vi "界面.vi"() -> ()   [LabVIEW 2021]
uses:
  <vilib>/Utility/file.llb/Write Delimited Spreadsheet (string).vi
panel:
  out "回答框":string
  in  "词数":dbl(slide)=50.38167938931298 scale=0.0..200.0
  in  "空白按钮":bool
  in  "发送":bool
  in  "输入框":string
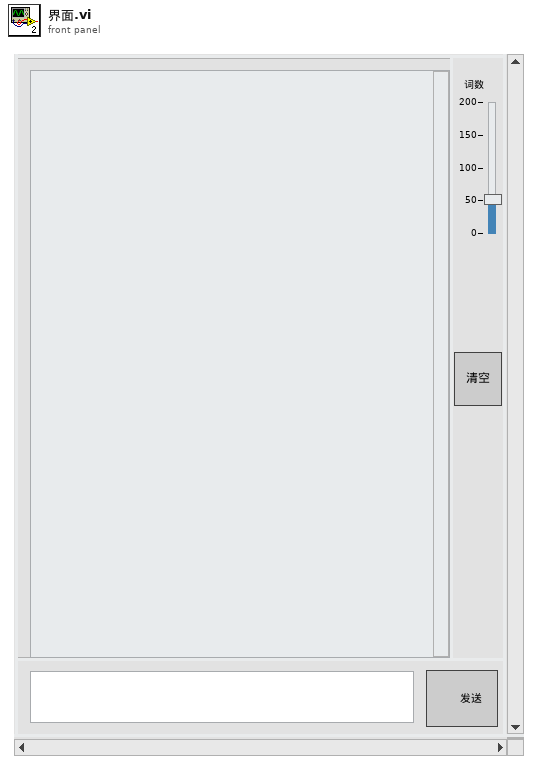
[diagram p1: front panel]
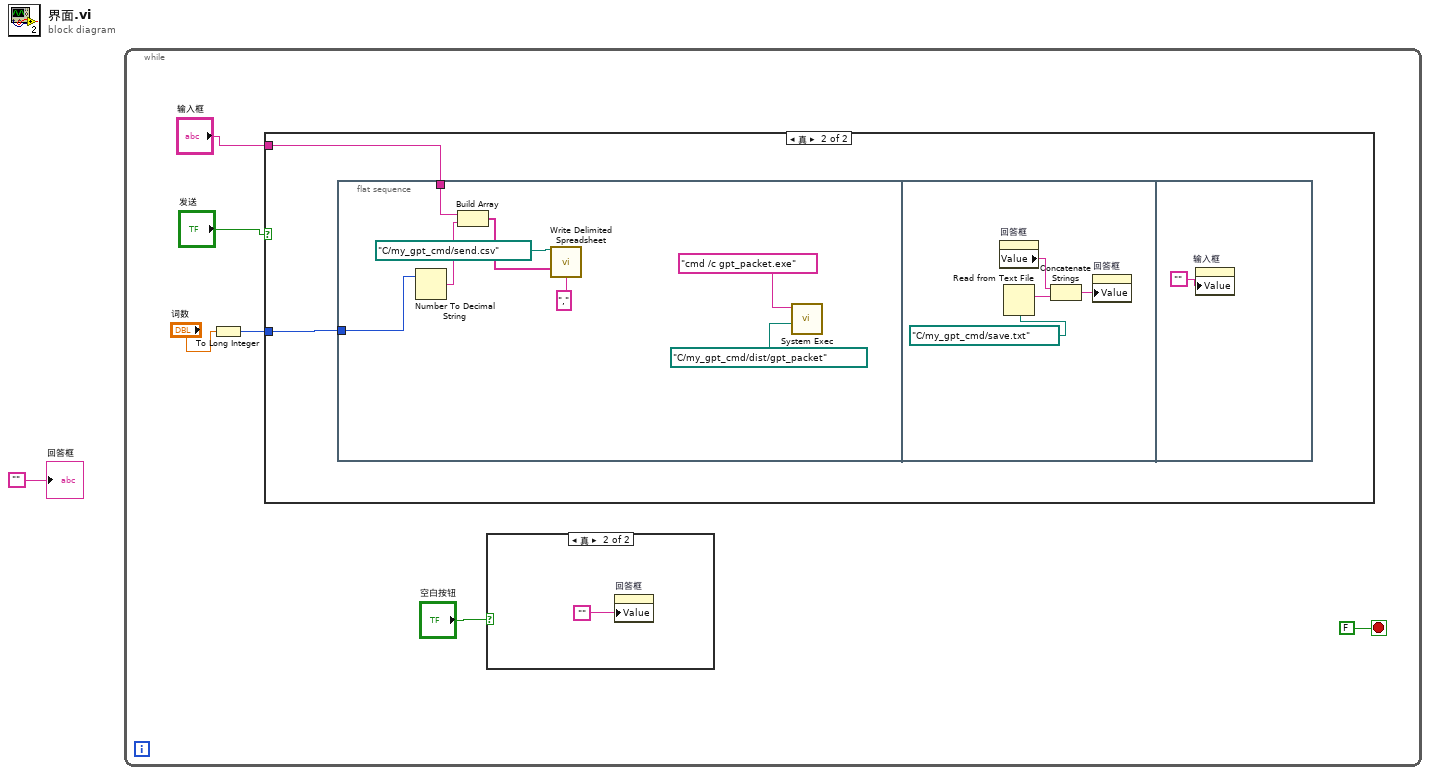
[diagram p0: block diagram]
diagram:
  n1 = while {
    stop <- FALSE stop-if-true
    n2 = To Long Integer(number="词数") -> (32bit integer=w2:i32)
    n3 = case shown="真" "发送" {
      tunnel: "输入框" -> [_ w10]
      tunnel: w2 -> [_ w9]
      frame False {
      }
      frame True {
        n4 = flat-sequence {
          tunnel: w10 -> [w17]
          tunnel: w9 -> [w18]
          frame #0 {
            n5 = Number To Decimal String(number=w18) -> (decimal integer string=w16:string)  [unwired: 1 in]
            n6 = Build Array(w17, w16) -> (w15:string[])
            n7 = call-poly <vilib>:"Write Delimited Spreadsheet.vi"("file path (dialog if empty)"=path "C:/my_gpt_cmd/send.csv", "1D data"=w15, "delimiter (\\t)"="," ("delimiter (\\t)")) -> ()  [unwired: 11 in, 2 out]
            n8 = call <vilib>:"System Exec.vi"("working directory"=path "C:/my_gpt_cmd/dist/gpt_packet", "command line"="cmd /c gpt_packet.exe") -> ()  [unwired: 6 in, 4 out]
          }
          frame #1 {
            n9 = property on="回答框" class="Str"() -> ("Value"=w20:string)  [unwired: 2 in, 2 out]
            n10 = Read from Text File(file (use dialog)=path "C:/my_gpt_cmd/save.txt" ("文件（使用对话框）")) -> (text=w22:string)  [unwired: 3 in, 3 out]
            n11 = Concatenate Strings(w20, w22) -> (w21:string)
            n12 = property on="回答框" class="Str"("Value"=w21) -> ()  [unwired: 2 in, 2 out]
          }
          frame #2 {
            n13 = property on="输入框" class="Str"("Value"="") -> ()  [unwired: 2 in, 2 out]
          }
        }
      }
    }
    n14 = case shown="真" "空白按钮" {
      frame False {
      }
      frame True {
        n15 = property on="回答框" class="Str"("Value"="") -> ()  [unwired: 2 in, 2 out]
      }
    }
  }
  "回答框" <- ""
